vi "Add Wrapper.vi"(11 "error in (no error)":errorcluster) -> (15 "error out":errorcluster)   [LabVIEW 2021, in "Converter.lvlib"]
uses:
  Converter.lvlib
  Path Functions/Path Functions.lvlib
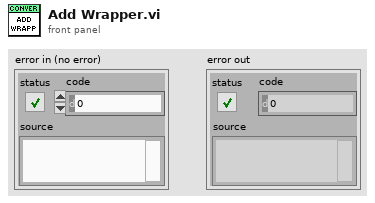
[diagram p1: front panel]
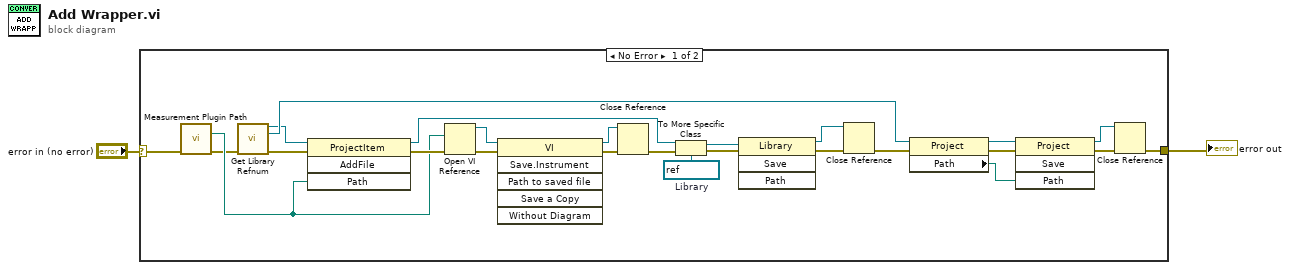
[diagram p0: block diagram]
diagram:
  n1 = case shown="No Error" "error in (no error)" {
    selector: "error in (no error)" -> [w4 w28]
    tunnel: [w24 w28] -> w2
    frame No Error {
      w15 = refnum<vi> refnum  # Library
      n2 = call "Measurement Plugin Path.vi"("error in (no error)"=w4) -> ("Wrapper Path"=w5:path, "error out"=w3:errorcluster)  [unwired: 2 in, 11 out]
      n3 = call "Get Library Refnum.vi"("error in (no error)"=w3) -> ("Library Refnum"=w16:refnum<vi>, "Project:Open"=w22:refnum<vi>, "error out"=w18:errorcluster)  [unwired: 12 in]
      n4 = invoke class="ProjectItem" method="AddFile"(reference=w16, error in=w18, "Path"=w5) -> (reference out=w12:refnum<vi>, error out=w7:errorcluster)  [unwired: 1 in, 2 out]
      n5 = Open VI Reference(vi path=w5, error in (no error)=w7) -> (vi reference=w8:refnum<vi>, error out=w6:errorcluster)  [unwired: 4 in]
      n6 = invoke class="VI" method="Save.Instrument"(reference=w8, error in=w6) -> (reference out=w9:refnum<vi>, error out=w10:errorcluster)  [unwired: 4 in, 4 out]
      n7 = Close Reference(reference=w9, error in (no error)=w10) -> (error out=w17:errorcluster)
      n8 = To More Specific Class(target class=w15, reference=w12, error in=w17) -> (specific class reference=w14:refnum<vi>, error out=w13:errorcluster)
      n9 = invoke class="Library" method="Save"(reference=w14, error in=w13) -> (reference out=w21:refnum<vi>, error out=w20:errorcluster)  [unwired: 2 in, 2 out]
      n10 = Close Reference(reference=w21, error in (no error)=w20) -> (error out=w19:errorcluster)
      n11 = property class="Project"(reference=w22, error in=w19) -> (reference out=w11:refnum<vi>, error out=w25:errorcluster, "Path"=w27:path)
      n12 = invoke class="Project" method="Save"(reference=w11, error in=w25, "Path"=w27) -> (reference out=w23:refnum<vi>, error out=w26:errorcluster)  [unwired: 1 in, 2 out]
      n13 = Close Reference(reference=w23, error in (no error)=w26) -> (error out=w24:errorcluster)
    }
    frame Error {
    }
  }
  "error out" <- w2
